vi "Coerce Wheel Angle.vi"(0 "Angle In":dbl) -> (1 "Wheel Angle":i8, 2 "Path Index":i32)   [LabVIEW 2010]
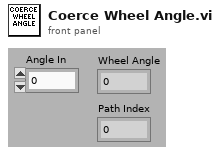
[diagram p1: front panel]
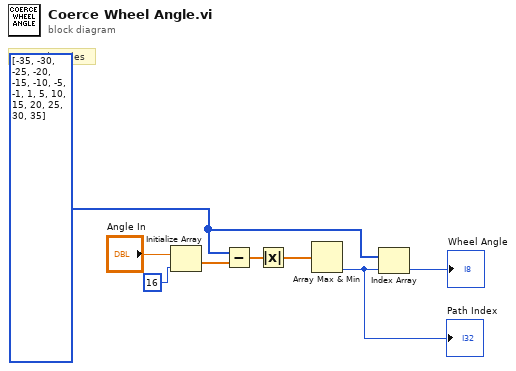
[diagram p0: block diagram]
diagram:
  w2 = i8[] [-35, -30, -25, -20, -15, -10, -5, -1, 1, 5, 10, 15, 20, 25, 30, 35]
  # "Coerced Angles"
  n1 = Initialize Array("Angle In", 16 ("dimension size")) -> (w6:dbl[])
  n2 = Subtract(x=w2, y=w6) -> (x-y=w5:dbl[])
  n3 = Absolute Value(x=w5) -> (abs(x)=w4:dbl[])
  n4 = Array Max & Min(array=w4) -> (min index (indices)=w3:i32)  [unwired: 3 out]
  "Path Index" <- w3
  n5 = Index Array(array=w2, index=w3) -> (element=→"Wheel Angle":i8)
